vi "Write CompactDAQ Settings.vi"(8 "error in (no error)":errorcluster, 10 "CompactDAQ Settings":cluster{"Allow Muxing?":bool}, 11 "CompactDAQ Configuration in":refnum<class "CompactDAQ Configuration.lvclass">) -> (0 "error out":errorcluster, 3 "CompactDAQ Configuration out":refnum<class "CompactDAQ Configuration.lvclass">)   [LabVIEW 2016, in "CompactDAQ Configuration.lvclass"]
uses:
  CompactDAQ Configuration.lvclass
  CompactDAQ Configuration.lvclass/CompactDAQ Configuration.ctl
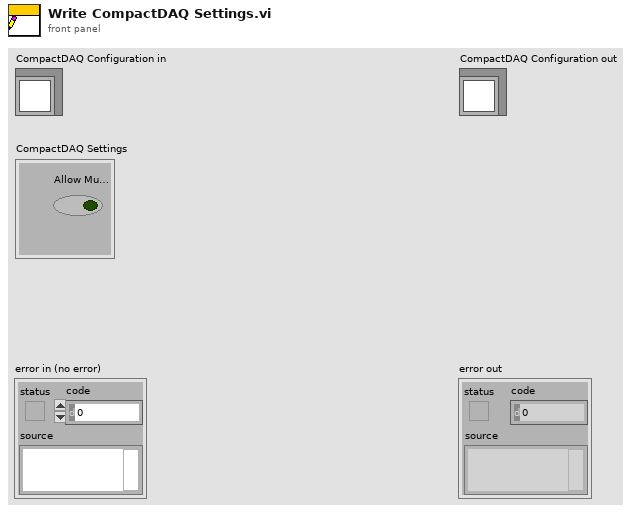
[diagram p1: front panel]
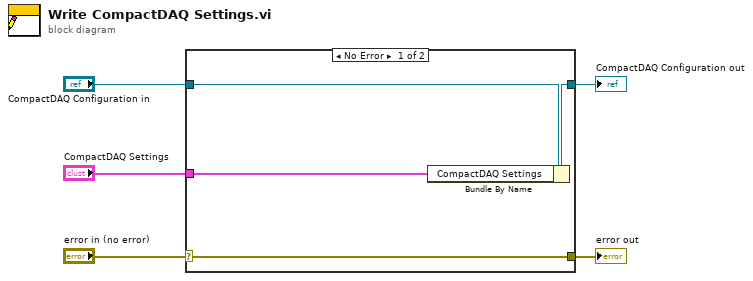
[diagram p0: block diagram]
diagram:
  n1 = case shown="No Error" "error in (no error)" {
    selector: "error in (no error)" -> [w9 w10]
    tunnel: [w9 w10] -> w4
    tunnel: [w7 w11] -> w2
    tunnel: "CompactDAQ Configuration in" -> [w8 w11]
    tunnel: "CompactDAQ Settings" -> [w6 _]
    frame No Error {
      n2 = Bundle By Name(cluster=w8, "CompactDAQ Settings"=w6) -> (w7:refnum<class "CompactDAQ Configuration.lvclass">)
    }
    frame Error {
    }
  }
  "error out" <- w4
  "CompactDAQ Configuration out" <- w2
